vi "HeartRateControl_SMC_New.vi"() -> ()   [LabVIEW 2013]
uses:
  <vilib>/Instr/_visa.llb/VISA Configure Serial Port (Instr).vi
panel:
  out "Volt2":dbl
  out "Volt":dbl
  out "TM":dbl
  in  "Target Heart Rate":dbl
  out "Torque [Nm]":dbl
  out "Cadence [rpm]":dbl
  out "Power [W]":dbl
  in  "file path (use dialog)":path
  out "Heart Rate [bpm]":u32
  out "Heart Rate [bpm]":dbl(knob) scale=0.0..220.0
  in  "VISA resource name":refnum<visa-resource-name>="COM1"
  out "Power [W]":dbl(slide) scale=0.0..250.0
  out "Cadence [rpm]":dbl(knob) scale=0.0..120.0
  out "Count":dbl
  out "Torque [Nm]":dbl(knob) scale=-250.0..250.0
  out "Torque [V]":dbl
  out "Sine":bool
  out "Cosine":bool
  in  "stop (F)":bool caption="Stop"
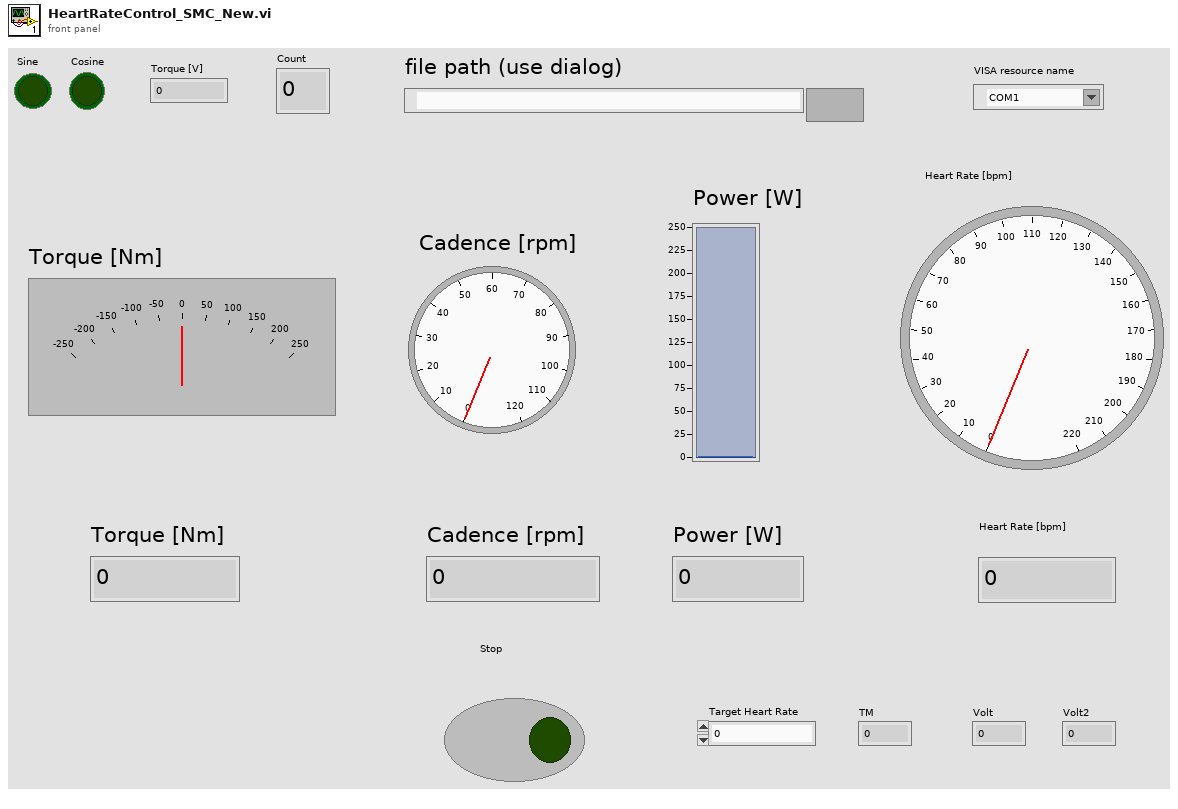
[diagram p1: front panel]
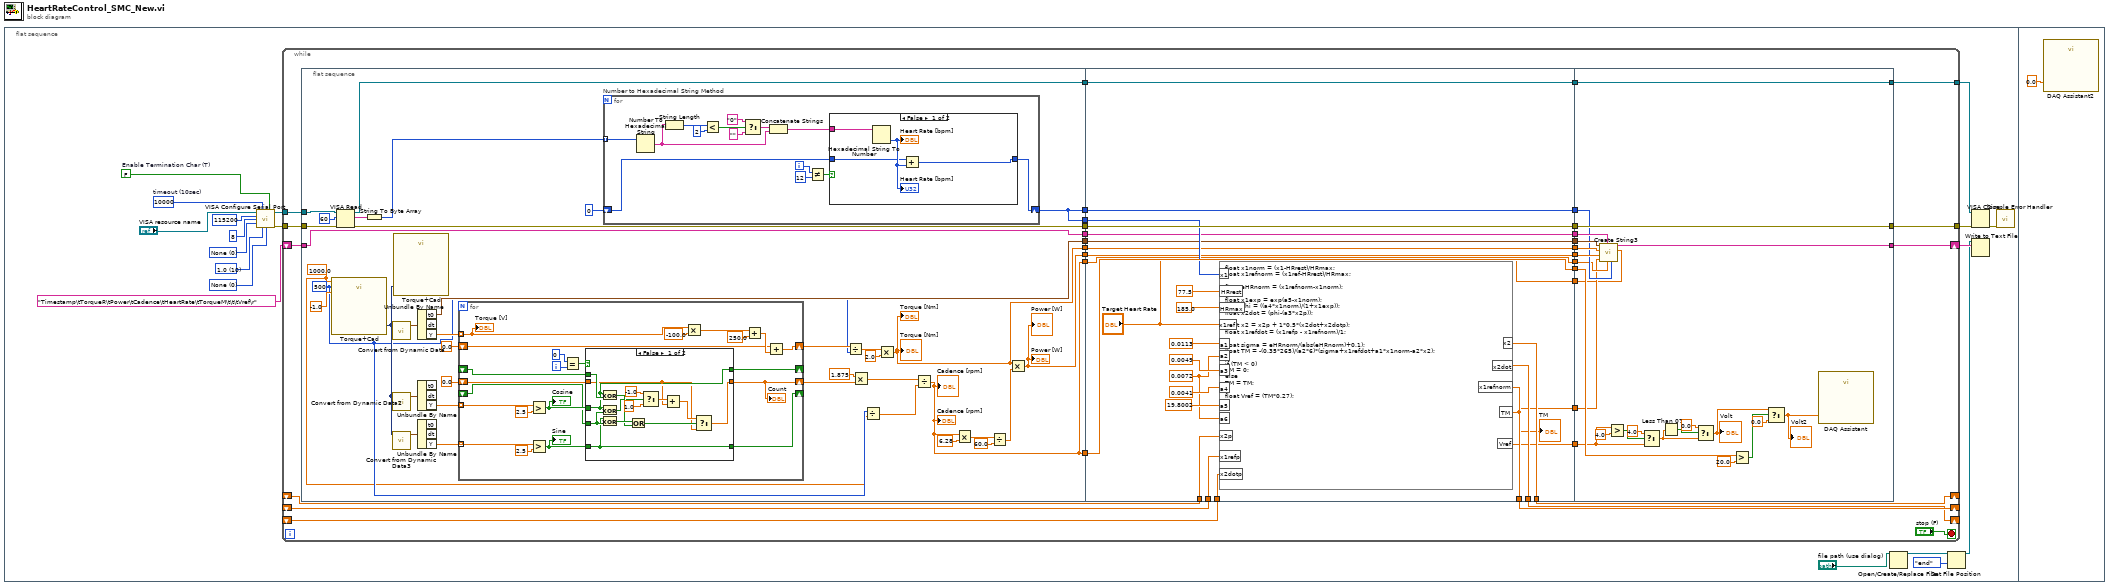
[diagram p0: block diagram]
diagram:
  n1 = flat-sequence {
    frame #0 {
      w14 = u16 0 items=["None"=0, "XON/XOFF"=1, "RTS/CTS"=2, "DTR/DSR"=4] ("flow control")
      w15 = u16 10 items=["1.0"=10, "1.5"=15, "2.0"=20] ("stop bits")
      w18 = u16 0 items=["None", "Odd", "Even", "Mark", "Space"] ("parity")
      w16 = FALSE  # Enable Termination Char (T)
      w17 = u32 10000  # timeout (10sec)
      n2 = call-poly "VISA Configure Serial Port"("VISA resource name"="VISA resource name", "timeout (10sec)"=w17, "Enable Termination\nChar (T)"=w16, "baud rate (9600)"=u32 115200, "data bits (8)"=u16 8, "parity (0:none)"=w18, "stop bits (10: 1 bit)"=w15, "flow control (0:none)"=w14) -> ("VISA resource name out"=w13:refnum<visa-resource-name>, "error out"=w12:errorcluster)  [unwired: 6 in]
      n3 = while {
        tunnel: w13 -> [w53]
        tunnel: w12 -> [w52]
        tunnel: [w51] -> w10
        tunnel: [w50] -> w9
        shift-right: [w49] -> w5
        shift-left: "Timestamp\tTorqueR\tPower\tCadence\tHeartRate\tTorqueM\t\t\tVref\r" ("String out") -> [w48]
        shift-right: [w25] -> _
        shift-left: _ -> [w44]
        shift-right: [w24] -> _
        shift-left: _ -> [w43]
        shift-right: [w23] -> _
        shift-left: _ -> [w38]
        stop <- "stop (F)" stop-if-true
        n4 = flat-sequence {
          tunnel: w53 -> [w70]
          tunnel: w52 -> [w69]
          tunnel: w48 -> [w62]
          tunnel: [w68] -> w47
          tunnel: [w67] -> w46
          tunnel: [w59] -> w45
          tunnel: [w58] -> w39
          tunnel: [w63] -> w36
          tunnel: [w62] -> w34
          tunnel: [w61] -> w32
          tunnel: [w60] -> w30
          tunnel: [w59] -> w28
          tunnel: [w58] -> w26
          tunnel: w47 -> [w175]
          tunnel: w46 -> [w174]
          tunnel: w45 -> [w170]
          tunnel: w44 -> [w159]
          tunnel: w43 -> [w157]
          tunnel: [w175] -> w42
          tunnel: [w174] -> w41
          tunnel: [w173] -> w40
          tunnel: w39 -> [w173]
          tunnel: w38 -> [w155]
          tunnel: [w169] -> w37
          tunnel: w36 -> [w169]
          tunnel: [w168] -> w35
          tunnel: w34 -> [w168]
          tunnel: [w167] -> w33
          tunnel: w32 -> [w167]
          tunnel: [w166] -> w31
          tunnel: w30 -> [w166]
          tunnel: [w165] -> w29
          tunnel: w28 -> [w165]
          tunnel: [w164] -> w27
          tunnel: w26 -> [w164]
          tunnel: [w160] -> w25
          tunnel: [w158] -> w24
          tunnel: [w156] -> w23
          tunnel: [w151] -> w22
          tunnel: [w152] -> w21
          tunnel: ["Target Heart Rate"] -> w20
          tunnel: [w185] -> w49
          tunnel: [w198] -> w50
          tunnel: [w199] -> w51
          tunnel: w42 -> [w199]
          tunnel: w41 -> [w198]
          tunnel: w40 -> [w188]
          tunnel: w37 -> [w184]
          tunnel: w35 -> [w183]
          tunnel: w33 -> [w182]
          tunnel: w31 -> [w181]
          tunnel: w29 -> [w180]
          tunnel: w27 -> [w179]
          tunnel: w22 -> [w177]
          tunnel: w21 -> [w178]
          tunnel: w20 -> [w176]
          frame #0 {
            w56 = 1000.0 ("rate")
            w57 = 500 ("number of samples")
            n5 = call "Torque+Cad"("rate"=w56, "number of samples"=w57, "timeout (s)"=-1.0) -> ("data"=w88:dynamicdata)  [unwired: 14 in, 2 out]
            n6 = VISA Read(VISA resource name=w70, byte count=u32 60 ("bytes to read"), error in (no error)=w69) -> (VISA resource name out=w68:refnum<visa-resource-name>, read buffer=w72:string, error out=w67:errorcluster)  [unwired: 1 out]
            n7 = String To Byte Array(string=w72) -> (unsigned byte array=w71:u8[])
            n8 = call "Convert from Dynamic Data"("Dynamic Data Type"=w88) -> ("Waveform"=w90:waveform(dbl))  [unwired: 3 in]
            n9 = call "Convert from Dynamic Data2"("Dynamic Data Type"=w88) -> ("Waveform"=w89:waveform(dbl))  [unwired: 3 in]
            n10 = call "Convert from Dynamic Data3"("Dynamic Data Type"=w88) -> ("Waveform"=w87:waveform(dbl))  [unwired: 3 in]
            n11 = call "Torque+Cad"("Signals"=w88) -> ()  [unwired: 16 in, 3 out]
            n12 = Unbundle By Name(w90) -> ("t0"=w63:timestamp, "Y"=w86:dbl[])  [unwired: 1 out]
            n13 = Unbundle By Name(w89) -> ("Y"=w85:dbl[])  [unwired: 2 out]
            n14 = Unbundle By Name(w87) -> ("Y"=w84:dbl[])  [unwired: 2 out]
            n15 = for {
              tunnel: w86 -> [w130] mode=indexing
              tunnel: w85 -> [w112] mode=indexing
              tunnel: w84 -> [w111] mode=indexing
              shift-right: [w123] -> _
              shift-left: _ -> [w119]
              shift-right: [w121] -> _
              shift-left: _ -> [w118]
              shift-right: [w117] -> w80
              shift-left: 0.0 -> [w116]
              shift-right: [w114] -> w79
              shift-left: 0.0 -> [w113]
              i -> [w126]
              n16 = Greater?(x=w112, y=2.5) -> (0:w120:bool)
              "Cosine" <- w120
              n17 = Greater?(x=w111, y=2.5) -> (0:w122:bool)
              "Sine" <- w122
              n18 = Equal?(x=0, y=w126) -> (x = y?=w124:bool)
              n19 = case shown="False" w124 {
                tunnel: [w135 w149] -> w123
                tunnel: w122 -> [w135 w149]
                tunnel: [w134 w148] -> w121
                tunnel: w120 -> [w134 w148]
                tunnel: w119 -> [w143 _]
                tunnel: w118 -> [w146 _]
                tunnel: [w136 w147] -> w117
                tunnel: w116 -> [w133 w147]
                frame False {
                  n20 = Exclusive Or(1:w146, 2:w134) -> (0:w144:bool)
                  n21 = Exclusive Or(1:w143, 2:w134) -> (0:w142:bool)
                  n22 = Exclusive Or(1:w143, 2:w135) -> (0:w145:bool)
                  n23 = Or(x=w145, y=w144) -> (x .or. y?=w141:bool)
                  n24 = Select(t=-1.0, s=w142, f=1.0) -> (s? t:f=w138:dbl)
                  n25 = Add(x=w138, y=w133) -> (x+y=w137:dbl)
                  n26 = Select(t=w137, s=w141, f=w133) -> (s? t:f=w136:dbl)
                }
                frame True {
                }
              }
              "Count" <- w117
              n27 = Multiply(x=w130, y=-100.0) -> (x*y=w128:dbl)
              n28 = Add(x=w128, y=250.0) -> (x+y=w115:dbl)
              n29 = Add(x=w113, y=w115) -> (x+y=w114:dbl)
              "Torque [V]" <- w130
            }
            n30 = for "Number to Hexadecimal String Method" {
              tunnel: w71 -> [w101] mode=indexing
              shift-right: [w93] -> w59
              shift-left: u32 0 -> [w92]
              i -> [w97]
              n31 = Number To Hexadecimal String(2:w101) -> (0:w98:string)  [unwired: 1 in]
              n32 = String Length(string=w98) -> (length=w105:i32)
              n33 = Less?(x=w105, y=2) -> (x < y?=w103:bool)
              n34 = Select(t="0", s=w103, f="") -> (s? t:f=w99:string)
              n35 = Concatenate Strings(w99, w98) -> (w94:string)
              n36 = Not Equal?(x=w97, y=12) -> (x != y?=w95:bool)
              n37 = case shown="False" w95 {
                tunnel: w94 -> [w109 _]
                tunnel: [w107 w110] -> w93
                tunnel: w92 -> [w106 w110]
                frame False {
                  n38 = Hexadecimal String To Number(string=w109) -> (number=w108:u32)  [unwired: 2 in, 1 out]
                  "Heart Rate [bpm]" <- w108
                  "Heart Rate [bpm]" <- w108
                  n39 = Add(x=w106, y=w108) -> (x+y=w107:u32)
                }
                frame True {
                }
              }
            }
            n40 = Divide(x=w79, y=w57) -> (x/y=w65:dbl)
            n41 = Multiply(x=1.875, y=w80) -> (x*y=w83:dbl)
            n42 = Divide(x=w57, y=w56) -> (x/y=w55:dbl)
            n43 = Multiply(x=w65, y=2.0) -> (x*y=w61:dbl)
            "Torque [Nm]" <- w61
            "Torque [Nm]" <- w61
            n44 = Divide(x=w83, y=w55) -> (x/y=w58:dbl)
            "Cadence [rpm]" <- w58
            "Cadence [rpm]" <- w58
            n45 = Multiply(x=w58, y=6.28) -> (x*y=w77:dbl)
            n46 = Divide(x=w77, y=60.0) -> (x/y=w75:dbl)
            n47 = Multiply(x=w61, y=w75) -> (x*y=w60:dbl)
            "Power [W]" <- w60
            "Power [W]" <- w60
          }
          frame #1 {
            w153 = 0.0072 ("input variable")
            n48 = formula code="float x1norm = (x1-HRrest)/HRmax;\nfloat x1refnorm = (x1ref-HRrest)/HRmax;\n\nfloat eHRnorm = (x1refnorm-x1norm);\n\nfloat x1exp = exp(a5-x1norm);\nfloat phi = ((a4*x1norm)/(1+x1exp));\nfloat x2dot = (phi-(a3*x2p));\n\nfloat x2 = x2p + 1*0.5*(x2dot+x2dotp);\nfloat x1refdot = (x1refp - x1refnorm)/1;\n\nfloat sigma = eHRnorm/(abs(eHRnorm)+0.1);\nfloat TM = -(0.35*265)/(a2*6)*(sigma+x1refdot+a1*x1norm-a2*x2);\n\nif (TM < 0)\nTM = 0;\nelse\nTM = TM;\n\nfloat Vref = (TM*0.27);"("x1"=w170, "HRrest"=77.5 ("y"), "HRmax"=185.0 ("y"), "x1ref"="Target Heart Rate", "a3"=0.0049 ("input variable"), "a4"=0.0041 ("input variable"), "a5"=19.8002 ("x"), "x2p"=w159, "x1refp"=w157, "x2dotp"=w155, "a2"=w153, "a1"=0.0113 ("input variable"), "a6"=w153) -> ("x2"=w160:dbl, "x2dot"=w156:dbl, "x1refnorm"=w158:dbl, "TM"=w152:dbl, "Vref"=w151:dbl)
            "TM" <- w152
          }
          frame #2 {
            n49 = call "Create String3.vi"("HRref"=w176, "Heart Rate"=w180, "Cadence"=w179, "String in"=w183, "Torque Motor"=w178, "Power"=w181, "Torque Rider"=w182, "t0"=w184) -> ("String out"=w185:string)  [unwired: 3 in]
            n50 = Greater?(x=w177, y=4.0) -> (0:w196:bool)
            n51 = Select(t=4.0, s=w196, f=w177) -> (s? t:f=w192:dbl)
            n52 = Less Than 0?(x=w192) -> (x < 0?=w194:bool)
            n53 = Select(t=0.0, s=w194, f=w192) -> (s? t:f=w186:dbl)
            "Volt" <- w186
            n54 = Greater?(x=w188, y=20.0) -> (0:w190:bool)
            n55 = Select(t=w186, s=w190, f=0.0) -> (s? t:f=w187:dbl)
            "Volt2" <- w187
            n56 = call "DAQ Assistant"("data"=w187) -> ()  [unwired: 17 in, 2 out]
          }
        }
      }
      n57 = Open/Create/Replace File(file path (use dialog)="file path (use dialog)") -> (refnum out=w3:refnum<file>)  [unwired: 5 in, 2 out]
      n58 = Set File Position(refnum=w3, from (0:start)=enum16{"start", "end", "current"}."end") -> (refnum out=w2:refnum<file>)  [unwired: 2 in, 1 out]
      n59 = VISA Close(VISA resource name=w10, error in (no error)=w9) -> (error out=w11:errorcluster)
      n60 = Write to Text File(file (use dialog)=w2, text=w5) -> ()  [unwired: 2 in, 3 out]
      n61 = call <vilib>:"Simple Error Handler.vi"("error in (no error)"=w11) -> ()  [unwired: 4 in, 5 out]
    }
    frame #1 {
      n62 = call "DAQ Assistant2"("data"=0.0) -> ()  [unwired: 17 in, 2 out]
    }
  }
